vi "Drag Force Set.vi"(8 "error in (no error)":errorcluster, 9 "Drag Coefficients (N/m)":T1={"kx (N/m)"=1.0, "ky (N/m)"=1.0, "kz (N/m)"=1.0} {"kx (N/m)" format="%.1f"; "ky (N/m)" format="%.1f"; "kz (N/m)" format="%.1f"}, 10 "Drag Force Toggles":T2={"X Drag"=TRUE, "Y Drag"=TRUE, "Z Drag"=TRUE}) -> (0 "error out":errorcluster)   [LabVIEW 2019, in "Haptic Prog Interface.lvlib"]
doc: "Enables and sets the drag coefficients of the pen for each directions (xyz).\n\n<b>Drag Force Toggles:</b> Accepts a cluster of 3 booleans, enabling the x, y, and z drag forces on the pen respectively.\n<b>Drag Coefficients:</b> Accepts a cluster of 3 numerical values, setting the x, y, and z drag coefficients respectively (note: F_drag = - k v, where k is the drag coefficient and v is the velocity)."
uses:
  Haptic Prog Interface.lvlib
  src/x64/Debug/Haptic Programming Interface.dll
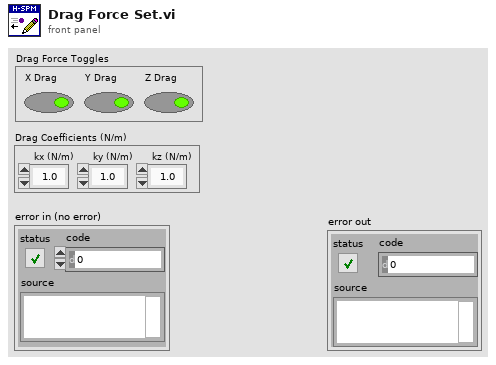
[diagram p1: front panel]
types:
  T1 = cluster{"kx (N/m)":dbl, "ky (N/m)":dbl, "kz (N/m)":dbl}
  T2 = cluster{"X Drag":bool, "Y Drag":bool, "Z Drag":bool}
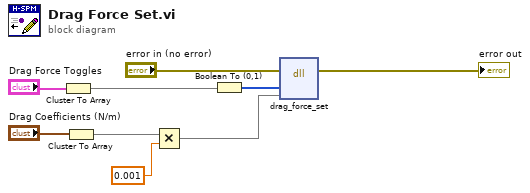
[diagram p0: block diagram]
diagram:
  n1 = Cluster To Array(cluster="Drag Force Toggles") -> (array=w5:bool[])
  n2 = Cluster To Array(cluster="Drag Coefficients (N/m)") -> (array=w3:dbl[])
  n3 = Multiply(x=w3, y=0.001) -> (x*y=w2:dbl[])
  n4 = Boolean To (0,1)(Boolean=w5) -> (0, 1=w7:i16[])
  n5 = dll-call lib="C:/Users/freem/Documents/GitHub/HapticSPM/Haptic-Programming-Interface/src/x64/Debug/Haptic Programming Interface.dll" fn="drag_force_set"(error in="error in (no error)", "toggle"=w7, "coeff"=w2) -> (error out=→"error out":errorcluster)  [unwired: 5 in, 1 out]
